vi "Patch data preview-Obtain TDMS ref.vi"(10 "Cycle number":i32, 11 "Register cluster":T1) -> (1 "Trial index":i32, 3 "TDMS ref":refnum<k34>)   [LabVIEW 2020]
uses:
  Typedefs/Patch viewer internal cluster.ctl
  <vilib>/vision/Image Controls.llb/IMAQ Image.ctl
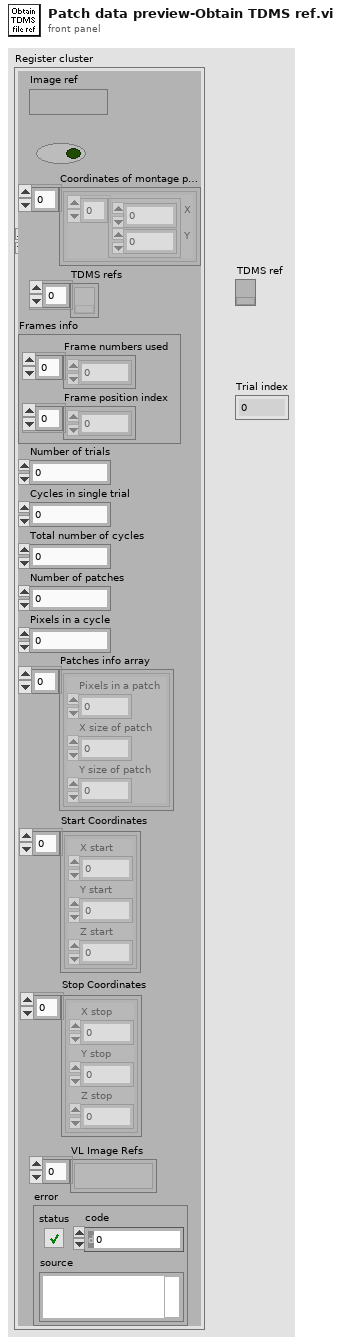
[diagram p1: front panel]
types:
  T1 = typedef "Patch viewer internal cluster.ctl" = cluster{"Image ref":T2, "Variable Length ?":bool, "Coordinates of montage positions":cluster{"X\n\nY":i32[]}[], "TDMS refs":refnum<k34>[], "Frames info":cluster{"Frame numbers used":i32[], "Frame position index":i32[]}, "Number of trials":i32, "Cycles in single trial":i32, "Total number of cycles":i32, "Number of patches":i32, "Pixels in a cycle":i32, "Patches info array":cluster{"Pixels in a patch":i32, "X size of patch":i32, "Y size of patch":i32}[], "Start Coordinates":cluster{"X start":i32, "Y start":i32, "Z start":i32}[], "Stop Coordinates":cluster{"X stop":i32, "Y stop":i32, "Z stop":i32}[], "VL Image Refs":T2[], "error":errorcluster}
  T2 = typedef "IMAQ Image.ctl" = refnum<image>
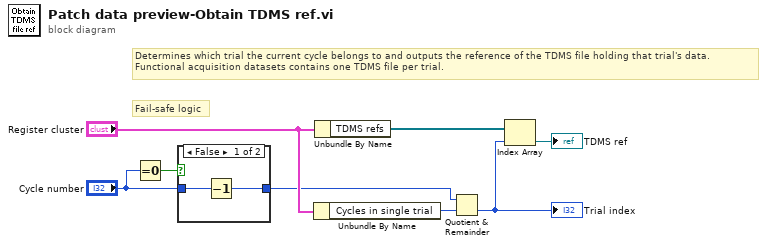
[diagram p0: block diagram]
diagram:
  # "Fail-safe logic"
  # "Determines which trial the current cycle belongs to and outputs the reference of the TDMS file holding that trial's data.\nFunctional acquisition datasets contains one TDMS file per trial."
  n1 = Equal To 0?(x="Cycle number") -> (x = 0?=w3:bool)
  n2 = case shown="False" w3 {
    tunnel: [w10 w11] -> w2
    tunnel: "Cycle number" -> [w9 w11]
    frame False {
      n3 = Decrement(x=w9) -> (x-1=w10:i32)
    }
    frame True {
    }
  }
  n4 = Unbundle By Name("Register cluster") -> ("Cycles in single trial"=w6:i32)
  n5 = Unbundle By Name("Register cluster") -> ("TDMS refs"=w8:refnum<k34>[])
  n6 = Quotient & Remainder(x=w2, y=w6) -> (floor(x/y)=w4:i32)  [unwired: 1 out]
  "Trial index" <- w4
  n7 = Index Array(array=w8, index=w4) -> (element=→"TDMS ref":refnum<k34>)
